vi "Response Characteristics.vi"(8 "Duration":u32, 9 "dt (s)":dbl, 10 "Setpoint":dbl, 11 "Process Variable":dbl) -> (0 "Recording":bool, 1 "Response":dbl[][](graph), 4 "% Overshot":dbl, 5 "Response Time (s)":dbl)   [LabVIEW 2011]
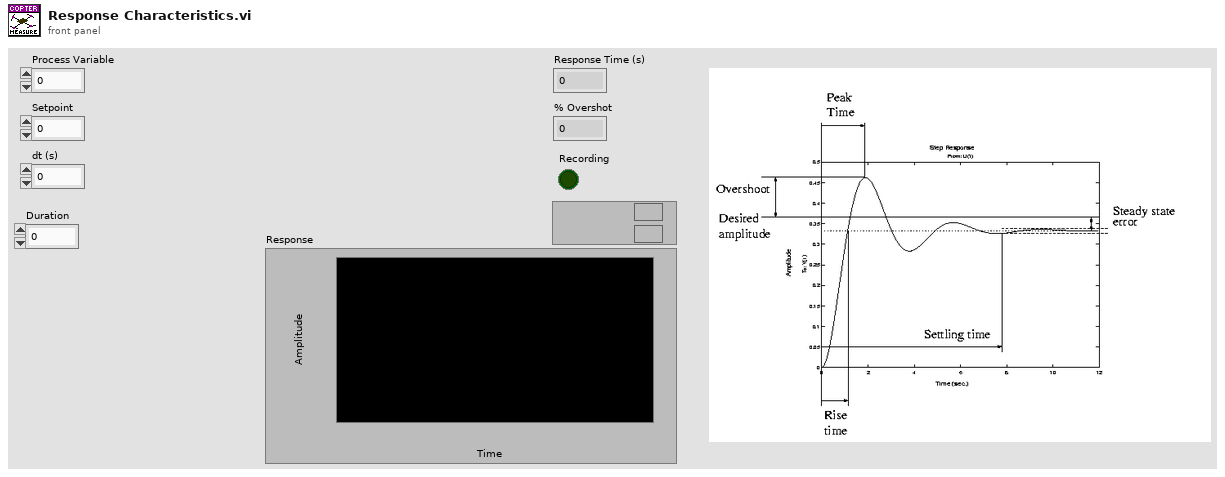
[diagram p1: front panel]
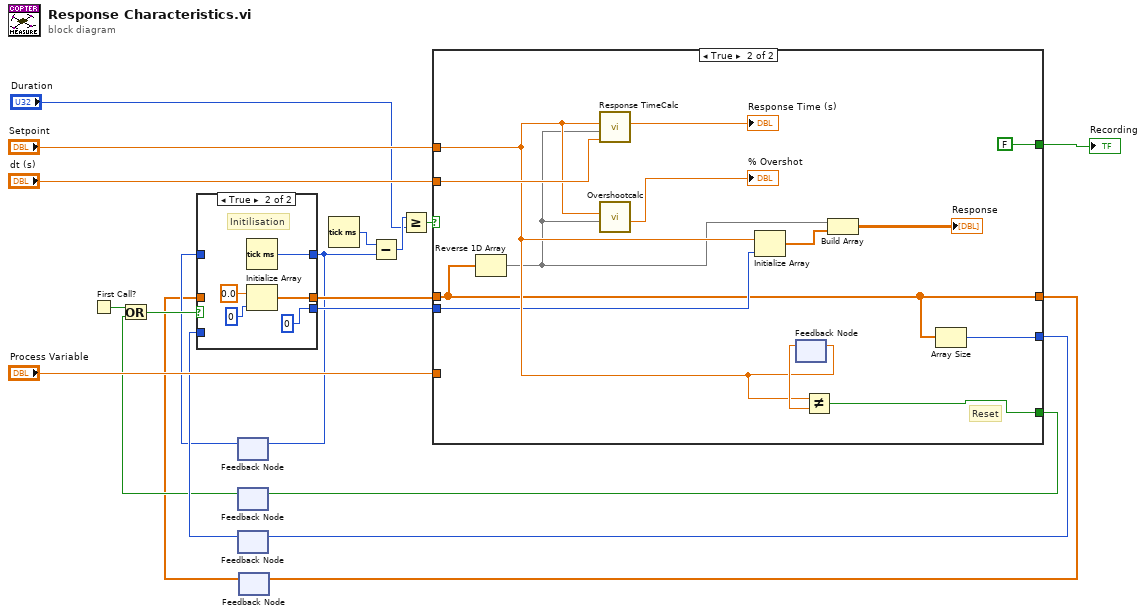
[diagram p0: block diagram]
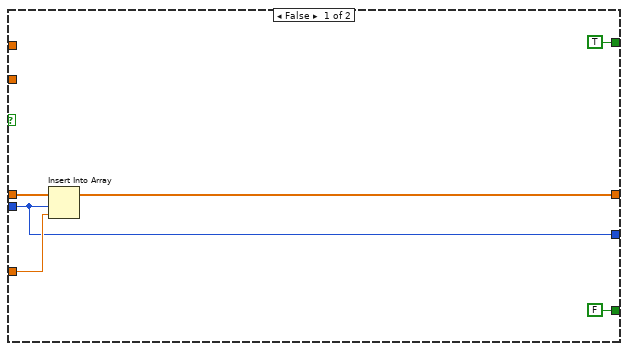
[diagram p2: hidden frame]
diagram:
  n1 = First Call?() -> (First Call?: T/F=w16:bool)
  n2 = feedback #1() -> (w10:u32)  [unwired: 1 in]
  n3 = feedback #2() -> (w13:bool)  [unwired: 1 in]
  n4 = Or(x=w16, y=w13) -> (x .or. y?=w15:bool)
  n5 = feedback #3() -> (w18:i32)  [unwired: 1 in]
  n6 = feedback #4() -> (w7:dbl[])  [unwired: 1 in]
  n7 = case shown="True" w15 {
    tunnel: [w22 w27] -> w17
    tunnel: [w21 0] -> w19
    tunnel: w18 -> [w21 _]
    tunnel: [w23 w24] -> w11
    tunnel: w10 -> [w23 _]
    tunnel: w7 -> [w22 _]
    frame False {
    }
    frame True {
      # "Initilisation"
      n8 = Tick Count (ms)() -> (millisecond timer value=w24:u32)
      n9 = Initialize Array(0.0 ("Process Variable 2"), 0 ("dimension size")) -> (w27:dbl[])
    }
  }
  n10 = feedback-in #1(w11) -> ()
  n11 = Tick Count (ms)() -> (millisecond timer value=w12:u32)
  n12 = Subtract(x=w12, y=w11) -> (x-y=w8:u32)
  n13 = Greater Or Equal?(x=w8, y="Duration") -> (x >= y?=w9:bool)
  n14 = case shown="True" w9 {
    tunnel: "Process Variable" -> [w34 _]
    tunnel: [w33 w37] -> w4
    tunnel: w19 -> [w31 w39]
    tunnel: w17 -> [w32 w37]
    tunnel: [FALSE w41] -> w14
    tunnel: "Setpoint" -> [_ w40]
    tunnel: "dt (s)" -> [_ w47]
    tunnel: [w31 w46] -> w3
    tunnel: [TRUE FALSE] -> w1
    frame False {
      n15 = Insert Into Array(array=w32, index=w31, new element=w34) -> (w33:dbl[])
    }
    frame True {
      # "Reset"
      n16 = Reverse 1D Array(array=w37) -> (reversed array=w36:dbl[])
      n17 = call "Response TimeCalc.vi"("dt (s)"=w47, "Response"=w36, "Setpoint"=w40) -> ("Response Time (s)"=→"Response Time (s)":dbl)  [unwired: 8 in]
      n18 = call "Overshootcalc.vi"("Response"=w36, "Setpoint"=w40) -> ("% Overshot"=→"% Overshot":dbl)  [unwired: 9 in]
      n19 = Initialize Array(w40, w39) -> (w38:dbl[])
      n20 = feedback #5() -> (w42:dbl)  [unwired: 1 in]
      n21 = feedback-in #5(w40) -> ()
      n22 = Not Equal?(x=w40, y=w42) -> (x != y?=w41:bool)
      n23 = Build Array(w36, w38) -> (→"Response":dbl[][])
      n24 = Array Size(array=w37) -> (size(s)=w46:i32)
    }
  }
  "Recording" <- w1
  n25 = feedback-in #2(w14) -> ()
  n26 = feedback-in #3(w3) -> ()
  n27 = feedback-in #4(w4) -> ()
